vi "LoadClassFromProject.vi"(8 "error in (no error)":errorcluster, 11 "PrjctItemRef":refnum<vi>) -> (0 "error out":errorcluster, 2 "object":refnum<class>, 3 "PrjctItemRef":refnum<vi>)   [LabVIEW 2020, in "CameraI2COUSB.lvlib" / "CameraDemo.lvclass"]
uses:
  CameraDemo.lvclass
  CameraDemo.lvclass/CameraDemo.ctl
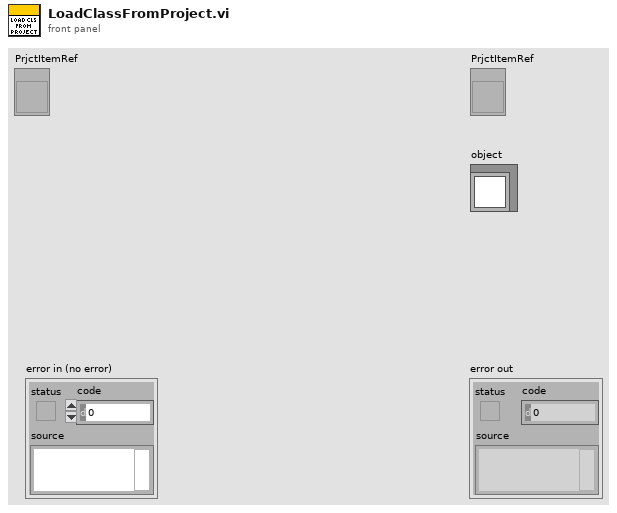
[diagram p1: front panel]
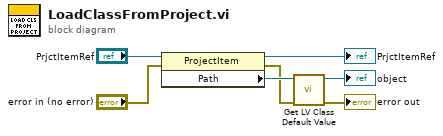
[diagram p0: block diagram]
diagram:
  n1 = property class="ProjectItem"(reference="PrjctItemRef", error in="error in (no error)") -> (reference out=→"PrjctItemRef":refnum<vi>, error out=w3:errorcluster, "Path"=w7:path)
  n2 = call <vilib>:"Get LV Class Default Value.vi"("error in (no error)"=w3, "class path"=w7) -> ("error out"=→"error out":errorcluster, "object"=→"object":refnum<class>)  [unwired: 8 in]
